vi "count_rising_edge.vi"(7 "reset":i32=1, 11 "target_reached":dbl) -> (3 "element 2":i32)   [LabVIEW 2015]
uses:
  BERTTA.dll
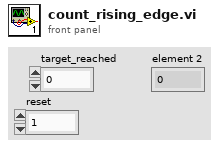
[diagram p1: front panel]
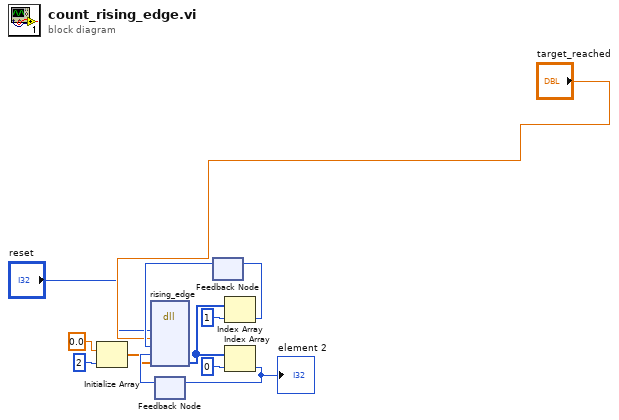
[diagram p0: block diagram]
diagram:
  n1 = Initialize Array(0.0 ("element"), 2 ("dimension size")) -> (w3:dbl[])
  n2 = feedback #1() -> (w8:i32)  [unwired: 1 in]
  n3 = feedback #2() -> (w12:i32)  [unwired: 1 in]
  n4 = dll-call lib="C:/Users/shresplab/OneDrive - Kemira Oyj/Documents/Visual Studio 2017/Projects/Bertta/BERTTA/x64/Debug/BERTTA.dll" fn="rising_edge"("reset"="reset", "input"="target_reached", "prev_input"=w12, "prev_count"=w8, "params"=w3) -> ("params"=w10:i32[])  [unwired: 8 in, 2 out]
  n5 = Index Array(array=w10, index=1) -> (element=w11:i32)
  n6 = feedback-in #2(w11) -> ()
  n7 = Index Array(array=w10, index=0) -> (element=w7:i32)
  "element 2" <- w7
  n8 = feedback-in #1(w7) -> ()
